vi "example test.vi"() -> ()   [LabVIEW 2013, in "Shared Library Module tests.lvlib"]
doc: "Platypus Framework 1.0.1.60\nNI Systems Engineering - National Instruments"
uses:
  Shared Library Module tests.lvlib
  configuration/Shared Library Module configuration.lvclass
  <vilib>/NI/Tag Bus Module Framework/channel/channel classification.ctl
  <vilib>/NI/Tag Bus/tag/Data Type.ctl
  execution/Shared Library Module runtime.lvclass
  <vilib>/NI/Tag Bus/dictionary/data dictionary.lvclass/data dictionary.ctl
  <vilib>/NI/Tag Bus/dictionary/lookup polymorphs/locate double.vi
  <vilib>/NI/Tag Bus/table/data polymorphs/write one/write Double.vi
  <vilib>/NI/Tag Bus/table/data polymorphs/read one/read Double.vi
  <vilib>/NI/Tag Bus/dictionary/search/find data index.vi
  <vilib>/NI/Tag Bus/dictionary/search/search string list.vi
  <vilib>/NI/Tag Bus/dictionary/tag not found.vi
  <vilib>/NI/Tag Bus Module Framework/channel/TBM channel.lvclass
  <vilib>/NI/Tag Bus/tag/tag descriptor.lvclass
  <vilib>/NI/Tag Bus/dictionary/data dictionary.lvclass
  <vilib>/NI/Tag Bus/table/data table.lvlib
panel:
  out "final error":errorcluster
  out "output error":errorcluster
  out "input error":errorcluster
  out "output lookup error":errorcluster
  out "no data written":bool
  out "input lookup error":errorcluster
  out "init error":errorcluster
  out "correct execution settings":bool
  out "serialization problem":errorcluster
  out "invalid configuration":errorcluster
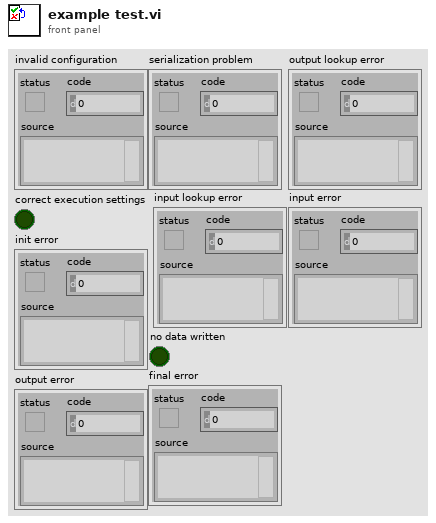
[diagram p1: front panel]
types:
  T1 = typedef "TBM channel.lvclass/channel classification.ctl" = enum16{"input data", "output data", "processing parameter", "processing result"}
  T2 = typedef "tag bus.lvlib/tag descriptor.lvclass/Data Type.ctl" = enum16{"Double", "Single", "I64", "I32", "I16", "I8", "U64", "U32", "U16", "U8", "Boolean", "String", "Array of Double", "Array of Single", "Array of I64", "Array of I32", "Array of I16", "Array of I8", "Array of U64", "Array of U32", "Array of U16", "Array of U8", "Array of Boolean", "Array of String"}
  T3 = typedef "TBM channel.lvclass/data tables.ctl" = cluster{"input data":T4, "processing parameter":T4, "processing result":T4, "output data":T4}
  T4 = typedef "tag bus.lvlib/dictionary table pair.ctl" = cluster{"data dictionary":refnum<class "data dictionary.lvclass">, "data table":T5}
  T5 = typedef "tag bus.lvlib/data table.lvlib/data table.ctl" = cluster{"Double":dbl[], "Single":sgl[], "I64":i64[], "I32":i32[], "I16":i16[], "I8":i8[], "U64":u64[], "U32":u32[], "U16":u16[], "U8":u8[], "Boolean":bool[], "String":string[], "Array of Double":cluster{"DBL Array":dbl[]}[], "Array of Single":cluster{"SGL Array":sgl[]}[], "Array of I64":cluster{"I64 Array":i64[]}[], "Array of I32":cluster{"I32 Array":i32[]}[], "Array of I16":cluster{"I16 Array":i16[]}[], "Array of I8":cluster{"I8 Array":i8[]}[], "Array of U64":cluster{"U64 Array":u64[]}[], "Array of U32":cluster{"U32 Array":u32[]}[], "Array of U16":cluster{"U16 Array":u16[]}[], "Array of U8":cluster{"U8 Array":u8[]}[], "Array of Boolean":cluster{"Boolean Array":bool[]}[], "Array of String":cluster{"String Array":string[]}[]}
  T6 = typedef "TBM module execution interface.lvclass/execution settings.ctl" = cluster{"reads inputs":bool, "processes data":bool, "writes outputs":bool}
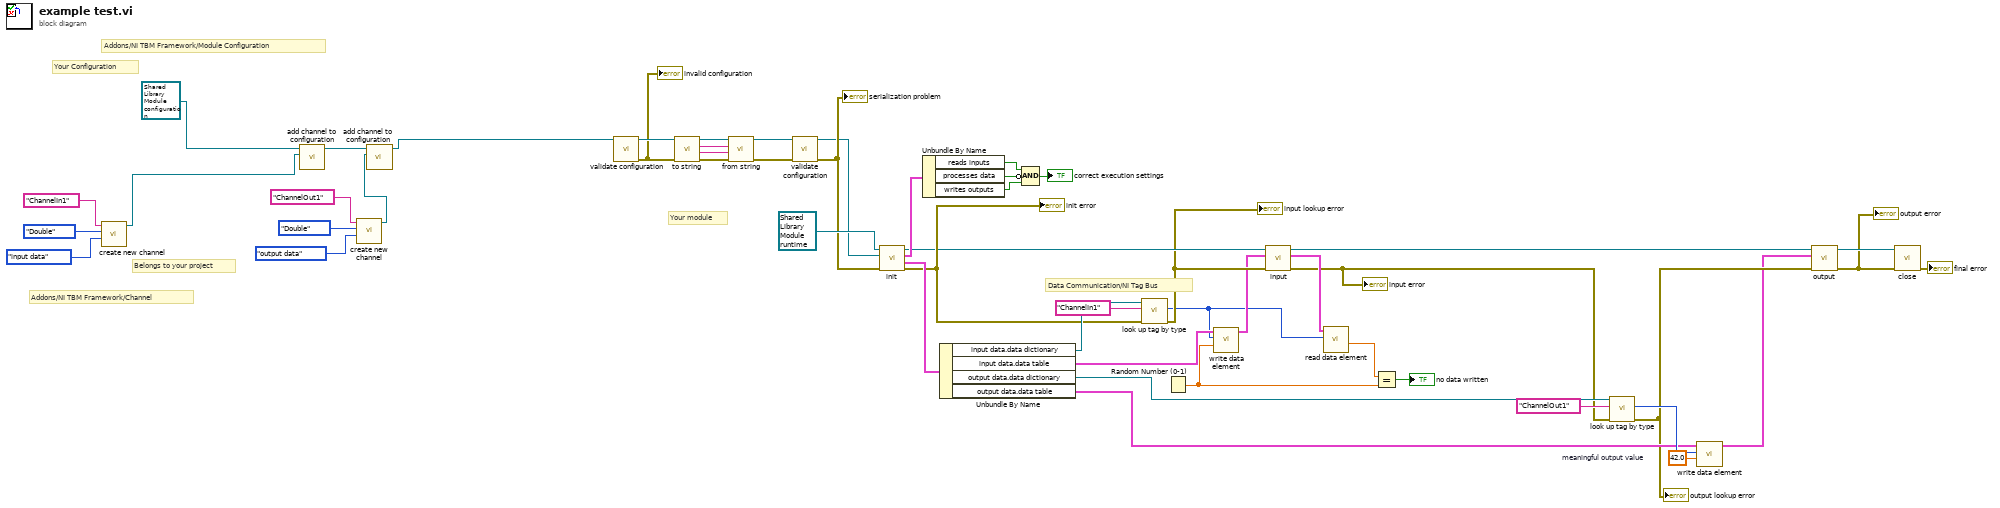
[diagram p0: block diagram]
diagram:
  w12 = 42.0  # meaningful output value
  # "Data Communication/NI Tag Bus"
  # "Your module"
  # "Your Configuration"
  # "Addons/NI TBM Framework/Module Configuration"
  # "Belongs to your project"
  # "Addons/NI TBM Framework/Channel"
  n1 = call <vilib>:"create new channel.vi"("channel classification"=channel_classification."input data", "data type"=Data_Type."Double", "channel name"="ChannelIn1") -> ("channel"=w1:refnum<class "TBM channel.lvclass">)  [unwired: 8 in]
  n2 = call "add channel to configuration.vi"("TBM channel in"=w1, "Shared Library Module configuration in"=refnum<class "Shared Library Module configuration.lvclass"> refnum ("tag bus configurable plugin module configuration")) -> ("Shared Library Module configuration out"=w4:refnum<class "Shared Library Module configuration.lvclass">)  [unwired: 8 in, 1 out]
  n3 = call <vilib>:"create new channel.vi"("channel classification"=channel_classification."output data", "data type"=Data_Type."Double", "channel name"="ChannelOut1") -> ("channel"=w2:refnum<class "TBM channel.lvclass">)  [unwired: 8 in]
  n4 = call "add channel to configuration.vi"("TBM channel in"=w2, "Shared Library Module configuration in"=w4) -> ("Shared Library Module configuration out"=w3:refnum<class "Shared Library Module configuration.lvclass">)  [unwired: 8 in, 1 out]
  n5 = call-dynamic "validate configuration.vi"("Shared Library Module configuration in"=w3) -> ("error out"=w45:errorcluster, "Shared Library Module configuration out"=w46:refnum<class "Shared Library Module configuration.lvclass">)  [unwired: 9 in]
  "invalid configuration" <- w45
  n6 = call-dynamic "to string.vi"("error in"=w45, "Shared Library Module configuration in"=w46) -> ("error out"=w41:errorcluster, "data"=w42:string, "version"=w43:string, "Shared Library Module configuration out"=w44:refnum<class "Shared Library Module configuration.lvclass">)  [unwired: 6 in]
  n7 = call-dynamic "from string.vi"("error in"=w41, "data"=w42, "version"=w43, "Shared Library Module configuration in"=w44) -> ("error out"=w39:errorcluster, "Shared Library Module configuration out"=w40:refnum<class "Shared Library Module configuration.lvclass">)  [unwired: 6 in]
  n8 = call-dynamic "validate configuration.vi"("error in"=w39, "Shared Library Module configuration in"=w40) -> ("error out"=w37:errorcluster, "Shared Library Module configuration out"=w36:refnum<class "Shared Library Module configuration.lvclass">)  [unwired: 8 in]
  "serialization problem" <- w37
  n9 = call-dynamic "init.vi"("error in"=w37, "TBM module configuration in"=w36, "Shared Library Module runtime in"=refnum<class "Shared Library Module runtime.lvclass"> refnum ("tag bus configurable plugin module")) -> ("error out"=w28:errorcluster, "data allocations"=w30:T3, "execution settings"=w35:T6, "Shared Library Module runtime out"=w25:refnum<class "Shared Library Module runtime.lvclass">)  [unwired: 5 in]
  "init error" <- w28
  n10 = Unbundle By Name(w35) -> ("reads inputs"=w32:bool, "processes data"=w34:bool, "writes outputs"=w33:bool)
  n11 = Unbundle By Name(w30) -> ("input data.data dictionary"=w29:refnum<class "data dictionary.lvclass">, "input data.data table"=w26:T5, "output data.data dictionary"=w17:refnum<class "data dictionary.lvclass">, "output data.data table"=w14:T5)
  n12 = Compound Arithmetic op=AND(w32, invert w34, w33) -> (→"correct execution settings":bool)
  n13 = call-poly <vilib>:"look up tag by type.vi"("error in"=w28, "name"="ChannelIn1" ("channel name"), "data dictionary in"=w29) -> ("error out"=w24:errorcluster, "index"=w21:i32)  [unwired: 6 in, 1 out]
  "input lookup error" <- w24
  n14 = Random Number (0-1)() -> (number: 0 to 1=w20:dbl)
  n15 = call-poly <vilib>:"write data element.vi"("value"=w20, "index"=w21, "data table in"=w26) -> ("data table out"=w23:T5)  [unwired: 8 in]
  n16 = call-dynamic "input.vi"("error in"=w24, "data table in"=w23, "Shared Library Module runtime in"=w25) -> ("error out"=w13:errorcluster, "data table out"=w22:T5, "Shared Library Module runtime out"=w10:refnum<class "Shared Library Module runtime.lvclass">)  [unwired: 6 in]
  "input error" <- w13
  n17 = call-poly <vilib>:"read data element.vi"("index"=w21, "data table in"=w22) -> ("value"=w19:dbl)  [unwired: 8 in, 1 out]
  n18 = Equal?(x=w19, y=w20) -> (x = y?=→"no data written":bool)
  n19 = call-poly <vilib>:"look up tag by type.vi"("error in"=w13, "name"="ChannelOut1" ("channel name"), "data dictionary in"=w17) -> ("error out"=w11:errorcluster, "index"=w15:i32)  [unwired: 6 in, 1 out]
  "output lookup error" <- w11
  n20 = call-poly <vilib>:"write data element.vi"("value"=w12, "index"=w15, "data table in"=w14) -> ("data table out"=w9:T5)  [unwired: 8 in]
  n21 = call-dynamic "output.vi"("error in"=w11, "data table in"=w9, "Shared Library Module runtime in"=w10) -> ("error out"=w7:errorcluster, "Shared Library Module runtime out"=w8:refnum<class "Shared Library Module runtime.lvclass">)  [unwired: 6 in, 1 out]
  "output error" <- w7
  n22 = call-dynamic "close.vi"("error in"=w7, "Shared Library Module runtime in"=w8) -> ("error out"=→"final error":errorcluster)  [unwired: 9 in]
